vi "Set Swerve Target.vi"(10 "Velocities":cluster{"LF":dbl, "LB":dbl, "RF":dbl, "RB":dbl}, 11 "Swerve drive motors":cluster{"LF":T2, "LB":T2, "RF":T2, "RB":T2}) -> ()   [LabVIEW 2020]
uses:
  <vilib>/Rock Robotics/WPI/MotorControl/WPI_MotorControlDeviceRef.ctl
  <vilib>/Rock Robotics/WPI/MotorControl/WPI_MotorControlType.ctl
  <vilib>/Rock Robotics/SystemInterfaces/DIO/FPGA_DIOPWMChannel.ctl
  <vilib>/Rock Robotics/WPI/PWM/WPI_PWMDeadband.ctl
  <vilib>/Rock Robotics/SystemInterfaces/DIO/FPGA_DIOChannel.ctl
  <vilib>/Rock Robotics/WPI/ThirdParty/Phoenix-LabVIEW/Motor Controller/Controls/CTRE_Phoenix_MotorControl_ControlMode.ctl
  <vilib>/Rock Robotics/WPI/ThirdParty/Phoenix-LabVIEW/Motor Controller/Get/CTRE_Phoenix_MotorController_GetSelectedSensorData.vi
panel:
  out "4":T1(graph)
  out "2":T1(graph)
  out "3":T1(graph)
  out "1":T1(graph)
  in  "F Drive":dbl
  in  "D Drive":dbl
  in  "I Drive":dbl
  in  "P Drive":dbl
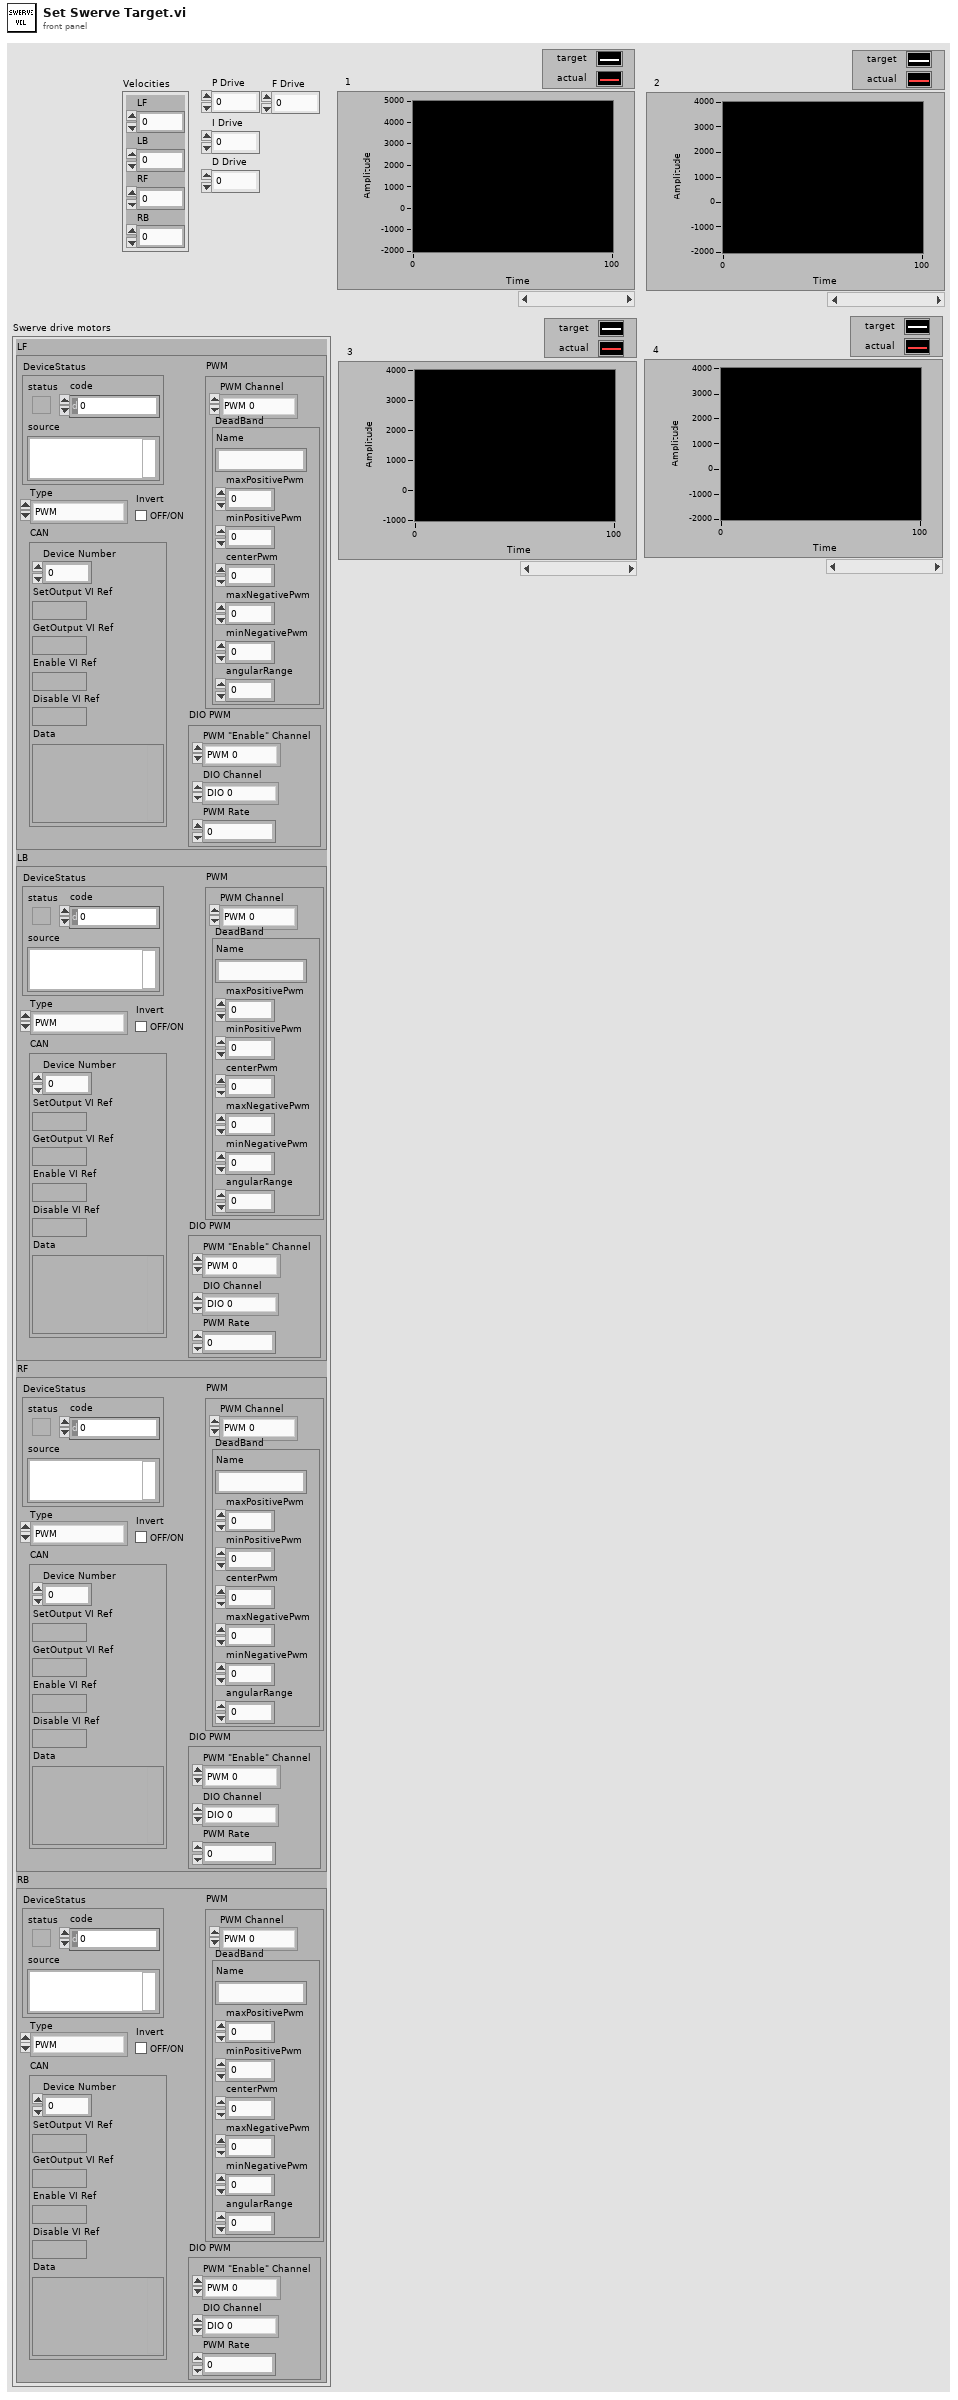
[diagram p1: front panel]
types:
  T1 = cluster{"Velocity (ticks/ms)":dbl, "Velocity (Raw Sensor Units per 100 ms)":i32}
  T2 = typedef "WPI_MotorControlDeviceRef.ctl" = cluster{"DeviceStatus":errorcluster, "Type":T3, "PWM":cluster{"PWM Channel":T4, "DeadBand":T5}, "CAN":cluster{"Device Number":u8, "SetOutput VI Ref":variant, "GetOutput VI Ref":variant, "Enable VI Ref":variant, "Disable VI Ref":variant, "Data":variant}, "Invert":bool, "DIO PWM":cluster{"PWM \"Enable\" Channel":T4, "DIOChannel":T6, "PWM Rate":dbl}}
  T3 = typedef "WPI_MotorControlType.ctl" = enum16{"PWM", "CAN", "DIO PWM"}
  T4 = typedef "FPGA_DIOPWMChannel.ctl" = enum8{"PWM 0", "PWM 1", "PWM 2", "PWM 3", "PWM 4", "PWM 5", "PWM 6", "PWM 7", "PWM 8", "PWM 9", "PWM MXP 0", "PWM MXP 1", "PWM MXP 2", "PWM MXP 3", "PWM MXP 4", "PWM MXP 5", "PWM MXP 6", "PWM MXP 7", "PWM MXP 8", "PWM MXP 9", "Invalid"}
  T5 = typedef "WPI_PWMDeadband.ctl" = cluster{"Name":string, "maxPositivePwm":i32, "minPositivePwm":i32, "centerPwm":i32, "maxNegativePwm":i32, "minNegativePwm":i32, "angularRange":u16}
  T6 = typedef "FPGA_DIOChannel.ctl" = enum8{"DIO 0", "DIO 1", "DIO 2", "DIO 3", "DIO 4", "DIO 5", "DIO 6", "DIO 7", "DIO 8", "DIO 9", "DIO MXP 0", "DIO MXP 1", "DIO MXP 2", "DIO MXP 3", "DIO MXP 4", "DIO MXP 5", "DIO MXP 6", "DIO MXP 7", "DIO MXP 8", "DIO MXP 9", "DIO MXP 10", "DIO MXP 11", "DIO MXP 12", "DIO MXP 13", "DIO MXP 14", "DIO MXP 15", "SPI Port CS1", "SPI Port CS2", "SPI Port CS3", "SPI Port MISO", "SPI Port MOSI", "Invalid"}
  T7 = typedef "CTRE_Phoenix_MotorControl_ControlMode.ctl" = u16
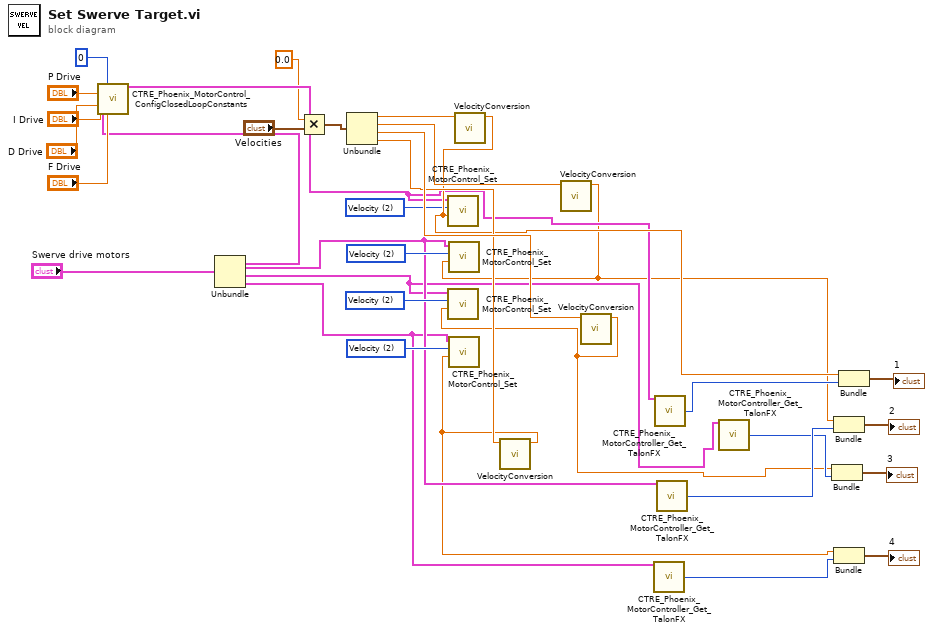
[diagram p0: block diagram]
diagram:
  w16 = T7 2 items=["PercentOutput"=0, "Position"=1, "Velocity"=2, "Current"=3, "Follower"=5, "MotionProfile"=6, "MotionMagic"=7, "MotionProfileArc"=10, "Disabled"=15] ("Control Mode")
  w17 = T7 2 items=["PercentOutput"=0, "Position"=1, "Velocity"=2, "Current"=3, "Follower"=5, "MotionProfile"=6, "MotionMagic"=7, "MotionProfileArc"=10, "Disabled"=15] ("Control Mode")
  w18 = T7 2 items=["PercentOutput"=0, "Position"=1, "Velocity"=2, "Current"=3, "Follower"=5, "MotionProfile"=6, "MotionMagic"=7, "MotionProfileArc"=10, "Disabled"=15] ("Control Mode")
  w19 = T7 2 items=["PercentOutput"=0, "Position"=1, "Velocity"=2, "Current"=3, "Follower"=5, "MotionProfile"=6, "MotionMagic"=7, "MotionProfileArc"=10, "Disabled"=15] ("Control Mode")
  n1 = Unbundle("Swerve drive motors") -> ("LF"=w21:T2, "LB"=w13:T2, "RF"=w11:T2, "RB"=w8:T2)
  n2 = call <vilib>:"CTRE_Phoenix_MotorControl_ConfigClosedLoopConstants.vi"("PhoenixMotorControlDevRef"=w21, "slotIdx"=0, "P"="P Drive", "I"="I Drive", "D"="D Drive", "F"="F Drive") -> ("PhoenixMotorControlDevRef"=w20:T2)  [unwired: 8 in, 1 out]
  n3 = Multiply(x=0.0 ("LF"), y="Velocities") -> (x*y=w2:cluster{"LF":dbl, "LB":dbl, "RF":dbl, "RB":dbl})
  n4 = Unbundle(w2) -> ("LF"=w33:dbl, "LB"=w32:dbl, "RF"=w31:dbl, "RB"=w30:dbl)
  n5 = call "VelocityConversion.vi"("Velocity (ft/s)"=w33) -> ("Velocity (ticks/ms)"=w23:dbl)  [unwired: 10 in]
  n6 = call <vilib>:"CTRE_Phoenix_MotorControl_Set.vi"("Output"=w23, "Control Mode"=w17, "PhoenixMotorControlDevRef"=w20) -> ()  [unwired: 7 in, 2 out]
  n7 = call "VelocityConversion.vi"("Velocity (ft/s)"=w30) -> ("Velocity (ticks/ms)"=w4:dbl)  [unwired: 10 in]
  n8 = call <vilib>:"CTRE_Phoenix_MotorControl_Set.vi"("Output"=w4, "Control Mode"=w18, "PhoenixMotorControlDevRef"=w8) -> ()  [unwired: 7 in, 2 out]
  n9 = call "VelocityConversion.vi"("Velocity (ft/s)"=w32) -> ("Velocity (ticks/ms)"=w12:dbl)  [unwired: 10 in]
  n10 = call <vilib>:"CTRE_Phoenix_MotorControl_Set.vi"("Output"=w12, "Control Mode"=w16, "PhoenixMotorControlDevRef"=w13) -> ()  [unwired: 7 in, 2 out]
  n11 = call "VelocityConversion.vi"("Velocity (ft/s)"=w31) -> ("Velocity (ticks/ms)"=w6:dbl)  [unwired: 10 in]
  n12 = call <vilib>:"CTRE_Phoenix_MotorControl_Set.vi"("Output"=w6, "Control Mode"=w19, "PhoenixMotorControlDevRef"=w11) -> ()  [unwired: 7 in, 2 out]
  n13 = call-poly <vilib>:"CTRE_Phoenix_MotorController_Get_TalonFX.vi"("PhoenixMotorControlDevRef"=w8) -> ("Velocity (Raw Sensor Units per 100 ms)"=w5:i32)  [unwired: 11 in, 3 out]
  n14 = call-poly <vilib>:"CTRE_Phoenix_MotorController_Get_TalonFX.vi"("PhoenixMotorControlDevRef"=w20) -> ("Velocity (Raw Sensor Units per 100 ms)"=w24:i32)  [unwired: 11 in, 3 out]
  n15 = call-poly <vilib>:"CTRE_Phoenix_MotorController_Get_TalonFX.vi"("PhoenixMotorControlDevRef"=w13) -> ("Velocity (Raw Sensor Units per 100 ms)"=w9:i32)  [unwired: 11 in, 3 out]
  n16 = call-poly <vilib>:"CTRE_Phoenix_MotorController_Get_TalonFX.vi"("PhoenixMotorControlDevRef"=w11) -> ("Velocity (Raw Sensor Units per 100 ms)"=w7:i32)  [unwired: 11 in, 3 out]
  n17 = Bundle("Velocity (ticks/ms)"=w6, "Velocity (Raw Sensor Units per 100 ms)"=w7) -> (→"3":T1)  [unwired: 1 in]
  n18 = Bundle("Velocity (ticks/ms)"=w12, "Velocity (Raw Sensor Units per 100 ms)"=w9) -> (→"2":T1)  [unwired: 1 in]
  n19 = Bundle("Velocity (ticks/ms)"=w4, "Velocity (Raw Sensor Units per 100 ms)"=w5) -> (→"4":T1)  [unwired: 1 in]
  n20 = Bundle("Velocity (ticks/ms)"=w23, "Velocity (Raw Sensor Units per 100 ms)"=w24) -> (→"1":T1)  [unwired: 1 in]
